vi "GetTotalDevNums.vi"(8 "错误输入（无错误）":errorcluster) -> (0 "错误输出":errorcluster, 3 "返回值":u8)   [LabVIEW 2014]
uses:
  ZXUTConfigMgr.dll
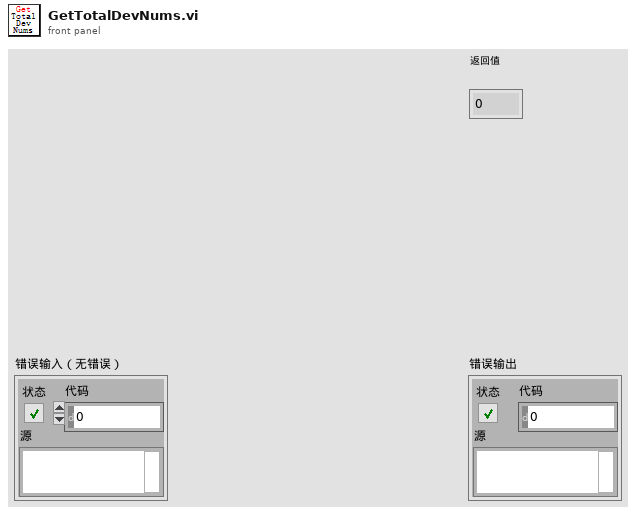
[diagram p1: front panel]
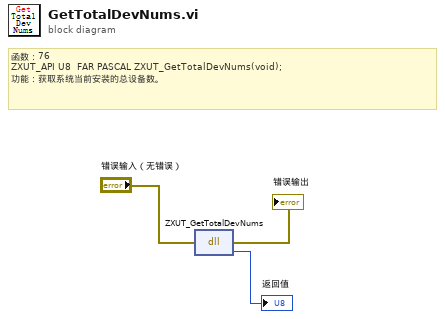
[diagram p0: block diagram]
diagram:
  # "函数：76\nZXUT_API U8\t\tFAR PASCAL ZXUT_GetTotalDevNums(void);\n功能：获取系统当前安装的总设备数。"
  n1 = dll-call lib="PTH2eabs D软件超声实时监测软件ZXUTAppDemo(华南理工V02.00)X86DllZXUTConfigMgr.dll" fn="ZXUT_GetTotalDevNums"(error in="错误输入（无错误）") -> (error out=→"错误输出":errorcluster, "返回值"=→"返回值":u8)  [unwired: 2 in, 1 out]
